vi "LC_Test.vi"() -> ()   [LabVIEW 2016]
panel:
  in  "Record Data":bool
  out "Record Status":string
  out "Array":dbl[](array[numeric])
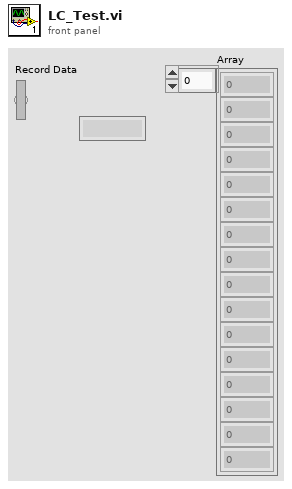
[diagram p1: front panel]
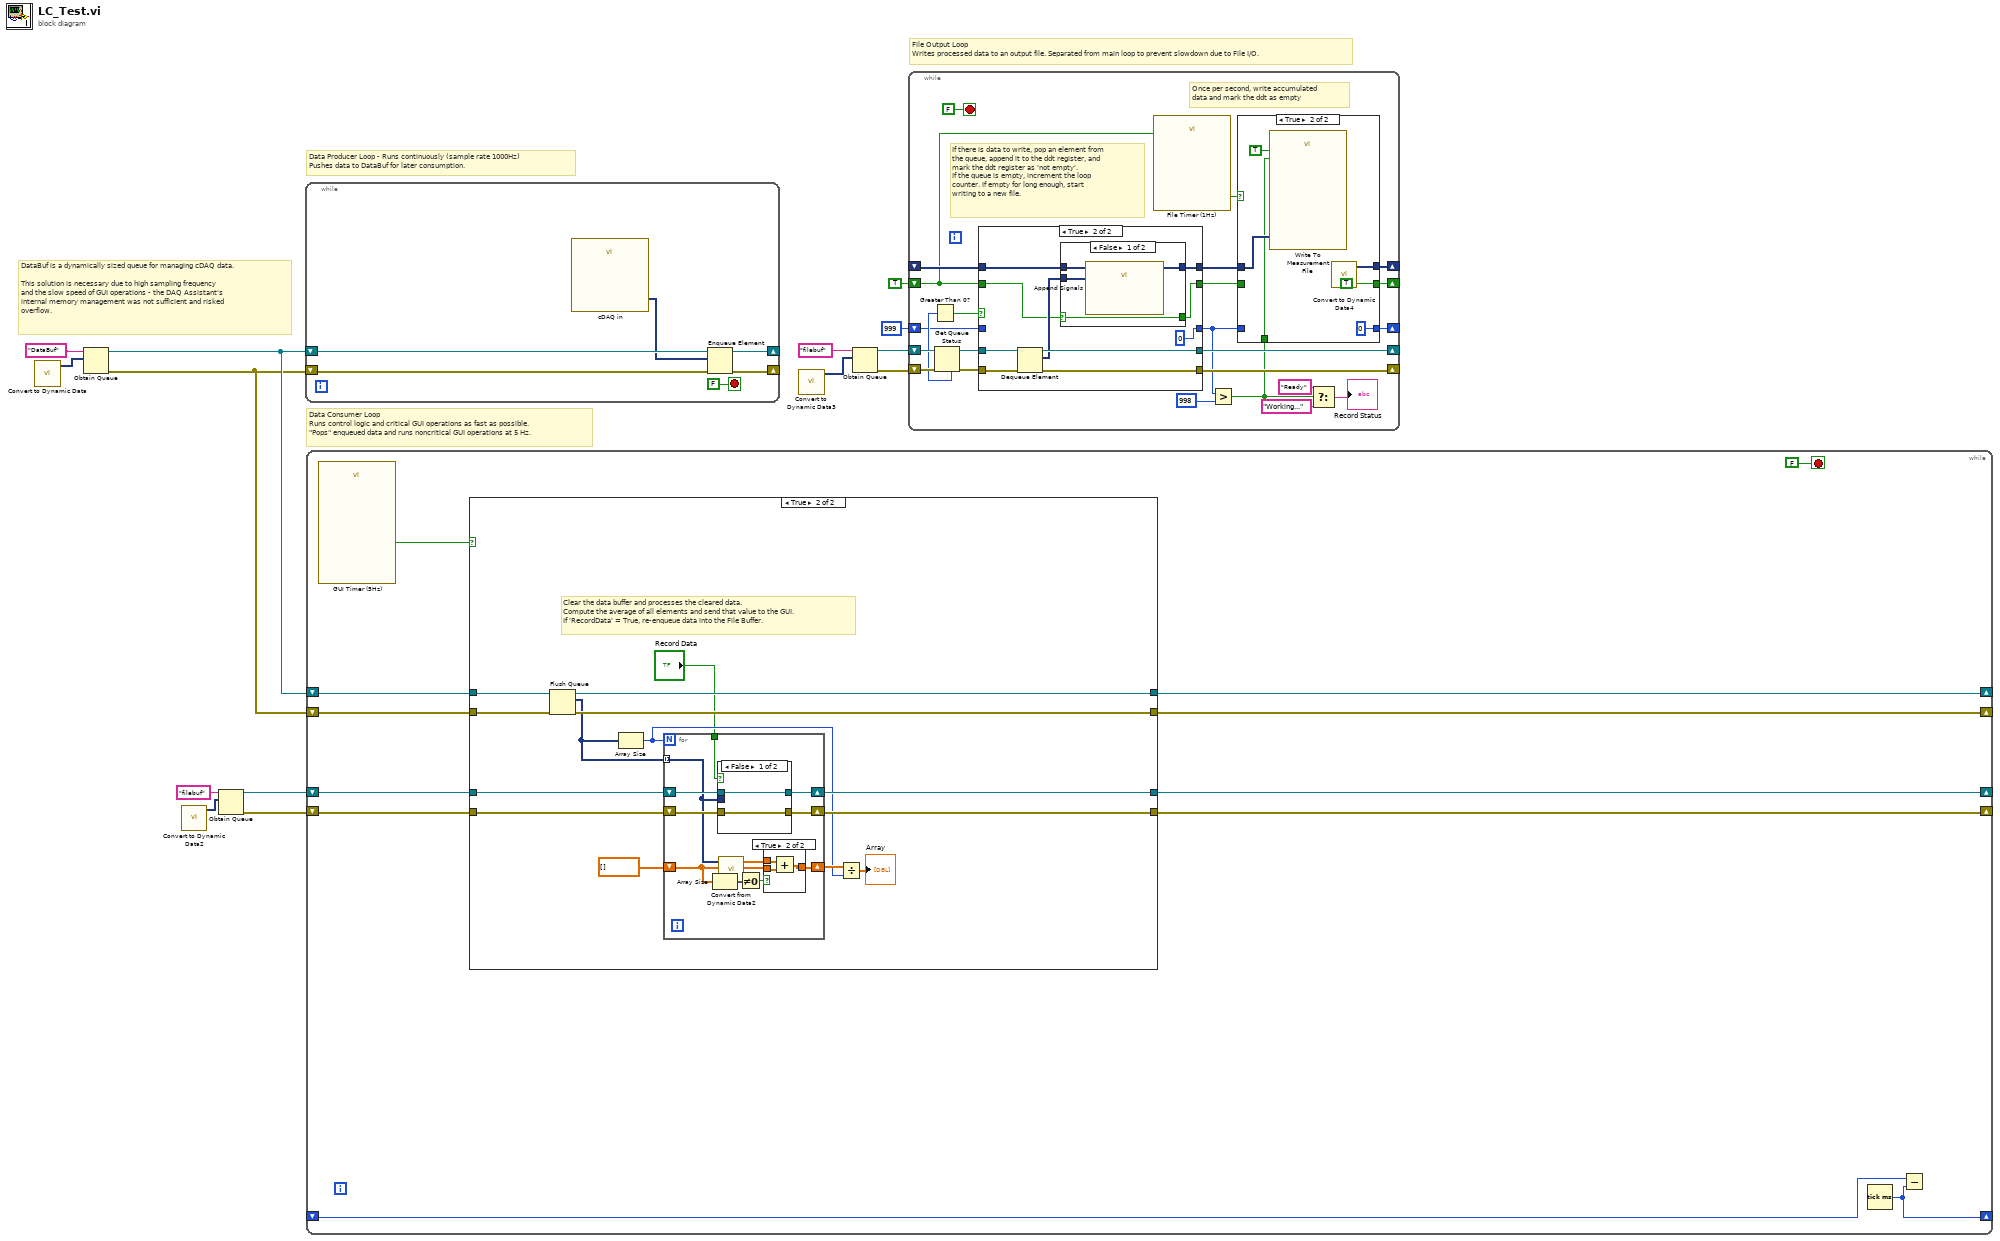
[diagram p0: block diagram]
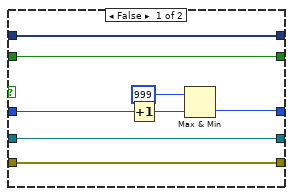
[diagram p3: hidden frame]
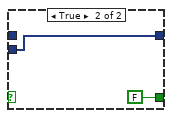
[diagram p4: hidden frame]
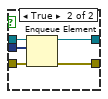
[diagram p6: hidden frame]
diagram:
  # "File Output Loop\nWrites processed data to an output file. Separated from main loop to prevent slowdown due to File I/O."
  # "Data Consumer Loop\nRuns control logic and critical GUI operations as fast as possible.\n\"Pops\" enqueued data and runs noncritical GUI operations at 5 Hz."
  # "Data Producer Loop - Runs continuously (sample rate 1000Hz)\nPushes data to DataBuf for later consumption."
  # "DataBuf is a dynamically sized queue for managing cDAQ data.\n\nThis solution is necessary due to high sampling frequency \nand the slow speed of GUI operations - the DAQ Assistant's\ninternal memory management was not sufficient and risked\noverflow."
  n1 = call "Convert to Dynamic Data"() -> ("Dynamic Data Type"=w13:dynamicdata)  [unwired: 4 in]
  n2 = Obtain Queue(name (unnamed)="DataBuf", element data type=w13) -> (queue out=w12:refnum<queue>, error out=w11:errorcluster)  [unwired: 3 in, 1 out]
  n3 = call "Convert to Dynamic Data2"() -> ("Dynamic Data Type"=w10:dynamicdata)  [unwired: 4 in]
  n4 = Obtain Queue(name (unnamed)="filebuf", element data type=w10) -> (queue out=w8:refnum<queue>, error out=w7:errorcluster)  [unwired: 3 in, 1 out]
  n5 = while {
    shift-right: [w17] -> _
    shift-left: w11 -> [w18]
    shift-right: [w19] -> _
    shift-left: w12 -> [w20]
    stop <- FALSE stop-if-true
    n6 = call "cDAQ in"() -> ("data"=w15:dynamicdata)  [unwired: 16 in, 3 out]
    n7 = Enqueue Element(queue=w20, element=w15, error in (no error)=w18) -> (queue out=w19:refnum<queue>, error out=w17:errorcluster)  [unwired: 1 in, 1 out]
  }
  n8 = while {
    shift-right: [w26] -> _
    shift-left: w12 -> [w28]
    shift-right: [w25] -> _
    shift-left: w11 -> [w27]
    shift-right: [w30] -> _
    shift-left: _ -> [w31]
    shift-right: [w22] -> _
    shift-left: w8 -> [w24]
    shift-right: [w21] -> _
    shift-left: w7 -> [w23]
    stop <- FALSE stop-if-true
    n9 = call "GUI Timer (5Hz)"() -> ("Time has Elapsed"=w29:bool)  [unwired: 12 in, 7 out]
    n10 = case shown="True" w29 {
      tunnel: w28 -> [w36 w50]
      tunnel: w27 -> [w35 w49]
      tunnel: [w36 w48] -> w26
      tunnel: [w35 w47] -> w25
      tunnel: w24 -> [w33 w45]
      tunnel: w23 -> [w34 w44]
      tunnel: [w33 w43] -> w22
      tunnel: [w34 w42] -> w21
      frame False {
      }
      frame True {
        # "Clear the data buffer and processes the cleared data.\nCompute the average of all elements and send that value to the GUI.\nIf 'RecordData' = True, re-enqueue data into the File Buffer."
        n11 = Flush Queue(queue=w50, error in (no error)=w49) -> (queue out=w48:refnum<queue>, remaining elements=w46:dynamicdata[], error out=w47:errorcluster)
        n12 = Array Size(array=w46) -> (size(s)=w38:i32)
        n13 = for {
          N: w38 -> [_]
          tunnel: w46 -> [w55] mode=indexing
          shift-right: [w59] -> w43
          shift-left: w45 -> [w61]
          shift-right: [w58] -> w42
          shift-left: w44 -> [w60]
          shift-right: [w53] -> w40
          shift-left: dbl[] [] -> [w52]
          tunnel: "Record Data" -> [w51]
          n14 = Array Size(array=w52) -> (size(s)=w56:i32)
          n15 = case shown="False" w51 {
            tunnel: w61 -> [w63 w68]
            tunnel: w60 -> [w62 w67]
            tunnel: [w63 w66] -> w59
            tunnel: [w62 w65] -> w58
            tunnel: w55 -> [_ w64]
            frame False {
            }
            frame True {
              n16 = Enqueue Element(queue=w68, element=w64, error in (no error)=w67) -> (queue out=w66:refnum<queue>, error out=w65:errorcluster)  [unwired: 1 in, 1 out]
            }
          }
          n17 = call "Convert from Dynamic Data2"("Dynamic Data Type"=w55) -> ("Array"=w54:dbl[])  [unwired: 3 in]
          n18 = Not Equal To 0?(x=w56) -> (x != 0?=w57:bool)
          n19 = case shown="True" w57 {
            tunnel: w54 -> [w69 w72]
            tunnel: w52 -> [_ w71]
            tunnel: [w69 w70] -> w53
            frame False {
            }
            frame True {
              n20 = Add(x=w72, y=w71) -> (x+y=w70:dbl[])
            }
          }
        }
        n21 = Divide(x=w40, y=w38) -> (x/y=→"Array":dbl[])
      }
    }
    n22 = Tick Count (ms)() -> (millisecond timer value=w30:u32)
    n23 = Subtract(x=w31, y=w30) -> ()  [unwired: 1 out]
  }
  n24 = call "Convert to Dynamic Data3"() -> ("Dynamic Data Type"=w5:dynamicdata)  [unwired: 4 in]
  n25 = Obtain Queue(name (unnamed)="filebuf", element data type=w5) -> (queue out=w4:refnum<queue>, error out=w3:errorcluster)  [unwired: 3 in, 1 out]
  n26 = while {
    shift-right: [w95] -> _
    shift-left: w3 -> [w87]
    shift-right: [w96] -> _
    shift-left: w4 -> [w88]
    shift-right: [w93] -> _
    shift-left: _ -> [w94]
    shift-right: [w92] -> _
    shift-left: TRUE -> [w81]
    shift-right: [w79] -> _
    shift-left: 999 -> [w80]
    stop <- FALSE stop-if-true
    # "If there is data to write, pop an element from\nthe queue, append it to the ddt register, and\nmark the ddt register as 'not empty'.\nIf the queue is empty, increment the loop\ncounter. If empty for long enough, start\nwriting to a new file."
    # "Once per second, write accumulated\ndata and mark the ddt as empty"
    n27 = Get Queue Status(queue=w88, error in (no error)=w87) -> (queue out=w90:refnum<queue>, error out=w89:errorcluster, # elements in queue=w85:i32)  [unwired: 1 in, 5 out]
    n28 = Greater Than 0?(x=w85) -> (x > 0?=w86:bool)
    n29 = case shown="True" w86 {
      tunnel: w90 -> [w112 w123]
      tunnel: w89 -> [w111 w122]
      tunnel: [w112 w121] -> w96
      tunnel: [w111 w120] -> w95
      tunnel: [w113 w119] -> w84
      tunnel: w94 -> [w113 w117]
      tunnel: w81 -> [w110 w116]
      tunnel: [w110 w115] -> w83
      tunnel: w80 -> [w109 _]
      tunnel: [w106 0] -> w75
      frame False {
        n30 = Increment(x=w109) -> (x+1=w108:i32)
        n31 = Max & Min(x=999, y=w108) -> (min(x,y)=w106:i32)  [unwired: 1 out]
      }
      frame True {
        n32 = Dequeue Element(queue=w123, error in (no error)=w122) -> (queue out=w121:refnum<queue>, element=w118:dynamicdata, error out=w120:errorcluster)  [unwired: 1 in, 1 out]
        n33 = case shown="False" w116 {
          selector: w116 -> [w124 _]
          tunnel: [w127 w129] -> w119
          tunnel: w118 -> [w126 w129]
          tunnel: w117 -> [w125 _]
          tunnel: [w124 FALSE] -> w115
          frame False {
            n34 = call "Append Signals"("Input Signal B"=w126, "Input Signal A"=w125) -> ("Appended Signals"=w127:dynamicdata)  [unwired: 8 in, 1 out]
          }
          frame True {
          }
        }
      }
    }
    n35 = call "File Timer (1Hz)"("Reset"=w81) -> ("Time has Elapsed"=w91:bool)  [unwired: 11 in, 7 out]
    n36 = Greater?(x=w75, y=998) -> (0:w74:bool)
    n37 = case shown="True" w91 {
      tunnel: [w98 w104] -> w93
      tunnel: [w99 TRUE] -> w92
      tunnel: w83 -> [w99 _]
      tunnel: w84 -> [w98 w103]
      tunnel: [w97 0] -> w79
      tunnel: w75 -> [w97 _]
      tunnel: w74 -> [_ w100]
      frame False {
      }
      frame True {
        n38 = call "Write To Measurement File"("Signals"=w103, "Enable"=TRUE, "new_file"=w100) -> ()  [unwired: 14 in, 3 out]
        n39 = call "Convert to Dynamic Data4"() -> ("Dynamic Data Type"=w104:dynamicdata)  [unwired: 4 in]
      }
    }
    n40 = Select(t="Ready", s=w74, f="Working...") -> (s? t:f=→"Record Status":string)
  }
